vi "FRC Color Processing RetroTape Example.vi"() -> ()   [LabVIEW 2019]
uses:
  <vilib>/Rock Robotics/Network Tables/NT Event Type.ctl
  <vilib>/Rock Robotics/Network Tables/Protocol Operations.ctl
  <vilib>/Rock Robotics/Network Tables/Field Data.ctl
  <vilib>/Rock Robotics/Network Tables/Field Type.ctl
  <vilib>/Rock Robotics/Network Tables/Sequence.ctl
  <vilib>/vision/NI_Vision_Development_Module.lvlib
panel:
  in  "Tab Control":enum32{"Mask", "Post Processed"}(tab)=enum."Post Processed"
  out "Mask":T1(plugin-control)
  in  "LED Color Range":T2={"Hue"={103.0, 151.0}, "Sat"={216.98804569244385, 255.0}, "Val"={201.0, 249.0}} {"Hue" scale=0.0..255.0 scale format="%#_3g"}
  in  "Color Mode":u16(ring)=2 items=["RGB", "HSL", "HSV", "HSI"]
  in  "Std Devs":cluster{"H":dbl, "S":dbl, "V":dbl}={"H"=6.0, "S"=6.0, "V"=6.0}
  out "Offset Angle":dbl=-14.437499999999998 format="%.1f"
  out "Fps Processing":dbl=128.6646791248816 format="%#.0f"
  out "Results":T3(array[cluster])=[{"diameter points"={"first point"={"x"=290.0, "y"=32.0}, "projected point"={"x"=196.0, "y"=45.0}}, "Normalized Center"={"x"=-0.24062499999999998, "y"=-0.7861111111111111}, "Overall Score"=94.92498623274359, "Area Score"=96.95566094203232, "Moment Score"=88.10546356152027, "Aspect Score"=99.71383419467818, "Distance (ft)"=13.68022905002843, "Upper Goal"=TRUE}] {"Normalized Center"."x" format="%#_2g"; "Normalized Center"."y" format="%#_2g"; "Overall Score" format="%#_2g"; "Distance (ft)" format="%#_3g"; "Area Score" format="%#_2g"; "Moment Score" format="%#_2g"; "Aspect Score" format="%#_2g"}
  in  "Exit":bool
  out "Loop Time":dbl=7.76519775390625 format="%0.2f"
  in  "Field of view":dbl=170.0 format="%#_13g"
  out "Processed":T1(plugin-control)
  in  "Client Name":string="Vision"
  in  "Update Time (ms)":i32=6
  in  "Server IP Address":string="roboRIO-141-FRC.local"
  # "Scores"
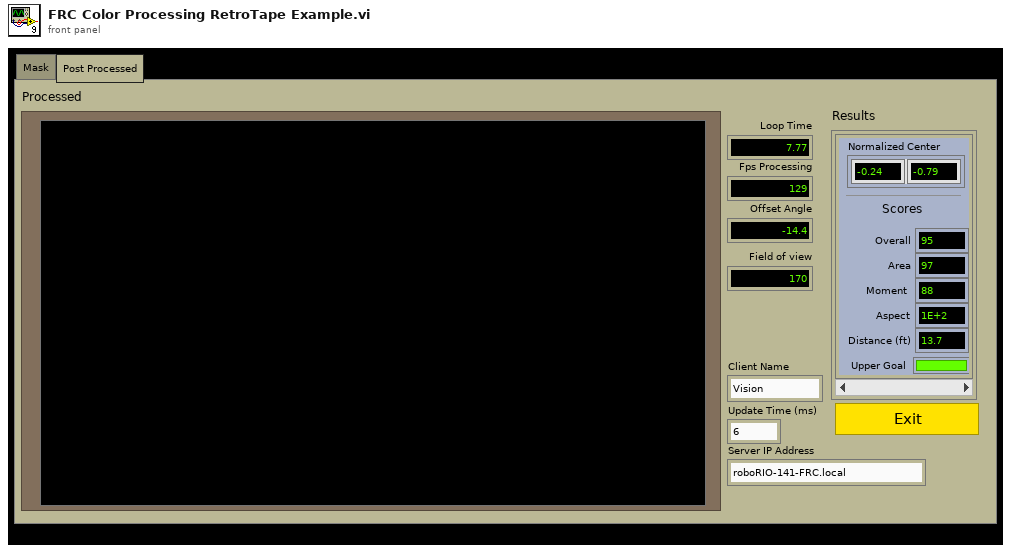
[diagram p1: front panel]
types:
  T1 = typedef "IMAQ Image.ctl" = refnum<image>
  T2 = cluster{"Hue":cluster{dbl, dbl}, "Sat":cluster{dbl, dbl}, "Val":cluster{dbl, dbl}}
  T3 = cluster{"diameter points":cluster{"first point":cluster{"x":dbl, "y":dbl}, "projected point":cluster{"x":dbl, "y":dbl}}, "Normalized Center":cluster{"x":dbl, "y":dbl}, "Overall Score":dbl, "Area Score":dbl, "Moment Score":dbl, "Aspect Score":dbl, "Distance (ft)":dbl, "Upper Goal":bool}[]
  T4 = typedef "NT Event Type.ctl" = cluster{"Operation":T5, "Name":string, "Field Value":T6}
  T5 = typedef "Protocol Operations.ctl" = enum16{"Unknown", "Keep Alive", "Client Hello", "Version not supported", "Server Hello Complete", "Assign", "Update", "No Op", "Server Hello", "Client Hello Complete", "Update Flags", "Delete Entry", "Delete All", "RPC Exec", "RPC Response"}
  T6 = typedef "Field Data.ctl" = cluster{"Dbl":dbl, "String":string, "Type":T7, "Boolean":bool, "Sequence #":T8, "Flags":u8}
  T7 = typedef "Field Type.ctl" = enum8{"Invalid", "Bool", "Numeric", "String", "Raw", "Boolean Array", "Numeric Array", "String Array", "RPC"}
  T8 = typedef "Sequence.ctl" = u16
  T9 = typedef "Image Type" = u32
  T10 = typedef "Particle Parameters" = i32
  T11 = cluster{cluster{dbl, dbl}, cluster{dbl, dbl}, cluster{dbl, dbl}}
  T12 = typedef "Target Fields.ctl" = cluster{"diameter points":cluster{"first point":cluster{"x":dbl, "y":dbl}, "projected point":cluster{"x":dbl, "y":dbl}}, "normalized center":cluster{"x":dbl, "y":dbl}, "Overall Score":dbl, "Area Score":dbl, "Moment Score":dbl, "Aspect Score":dbl, "Distance (ft)":dbl, "Upper Goal":bool}
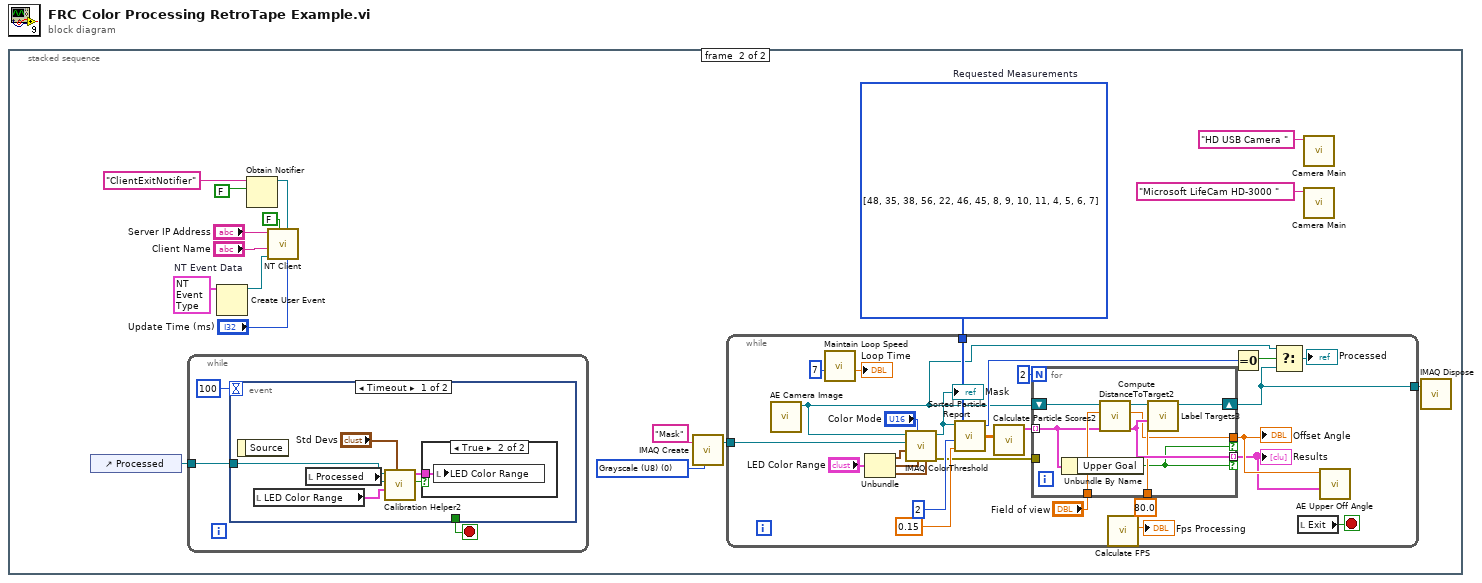
[diagram p0: block diagram]
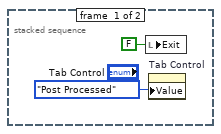
[diagram p2: hidden frame]
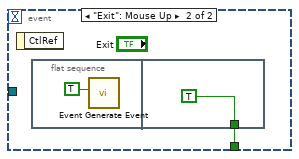
[diagram p4: hidden frame]
diagram:
  n1 = stacked-sequence {
    frame #0 {
      n2 = local write "Exit"(FALSE ("Exit")) -> ()
      n3 = property on="Tab Control" class="TabCtl (strict)"("Value"=enum32{"Mask", "Post Processed"}."Post Processed" ("Tab Control")) -> ()  [unwired: 2 in, 2 out]
    }
    frame #1 {
      w14 = T4 {"Operation"=enum."Assign", "Name"="", "Field Value"={"Dbl"=0.0, "String"="kjn", "Type"=enum."String", "Boolean"=FALSE, "Sequence #"=0, "Flags"=0}}  # NT Event Data
      w18 = T9 0 items=["Grayscale (U8)", "Grayscale (I16)", "Grayscale (SGL)", "Complex (CSG)", "RGB (U32)", "HSL (U32)", "RGB (U64)", "Grayscale (U16)"] ("Image Type")
      w19 = T10[] [48, 35, 38, 56, 22, 46, 45, 8, 9, 10, 11, 4, 5, 6, 7] items=["Center of Mass X", "Center of Mass Y", "First Pixel X", "First Pixel Y", "Bounding Rect Left", "Bounding Rect Top", "Bounding Rect Right", "Bounding Rect Bottom", "Max Feret Diameter Start X", "Max Feret Diameter Start Y", "Max Feret Diameter End X", "Max Feret Diameter End Y", "Max Horiz. Segment Length Left", "Max Horiz. Segment Length Right", "Max Horiz. Segment Length Row", "-", "Bounding Rect Width", "Bounding Rect Height", "Bounding Rect Diagonal", "Perimeter", "Convex Hull Perimeter", "Holes' Perimeter", "Max Feret Diameter", "Equivalent Ellipse Major Axis", "Equivalent Ellipse Minor Axis", "Equivalent Ellipse Minor Axis (Feret)", "Equivalent Rect Long Side", "Equivalent Rect Short Side", "Equivalent Rect Diagonal", "Equivalent Rect Short Side (Feret)", "Average Horiz. Segment Length", "Average Vert. Segment Length", "Hydraulic Radius", "Waddel Disk Diameter", "-", "Area", "Holes' Area", "Particle & Holes' Area", "Convex Hull Area", "Image Area", "-", "Number of Holes", "Number of Horiz. Segments", "Number of Vert. Segments", "-", "Orientation", "Max Feret Diameter Orientation", "-", "% Area/Image Area", "% Area/(Particle & Holes' Area)", "Ratio of Equivalent Ellipse Axes", "Ratio of Equivalent Rect Sides", "-", "Elongation Factor", "Compactness Factor", "Heywood Circularity Factor", "Type Factor", "-", "Sum X", "Sum Y", "Sum XX", "Sum XY", "Sum YY", "Sum XXX", "Sum XXY", "Sum XYY", "Sum YYY", "-", "Moment of Inertia XX", "Moment of Inertia XY", "Moment of Inertia YY", "Moment of Inertia XXX", "Moment of Inertia XXY", "Moment of Inertia XYY", "Moment of Inertia YYY", "Norm. Moment of Inertia XX", "Norm. Moment of Inertia XY", "Norm. Moment of Inertia YY", "Norm. Moment of Inertia XXX", "Norm. Moment of Inertia XXY", "Norm. Moment of Inertia XYY", "Norm. Moment of Inertia YYY", "Hu Moment 1", "Hu Moment 2", "Hu Moment 3", "Hu Moment 4", "Hu Moment 5", "Hu Moment 6", "Hu Moment 7"]  # Requested Measurements
      n4 = control-ref of="Processed"() -> (w3:refnum<vi>)
      n5 = while {
        tunnel: w3 -> [w22]
        stop <- w21 stop-if-true
        n6 = event shown="[0] Timeout" {
          selector: _ -> [_ _]
          dyn-events: _ -> [_ _]
          timeout: 100 -> [_ _]
          tunnel: w22 -> [w24 _]
          tunnel: [_ w30] -> w21
          event Timeout {
            n7 = event-data() -> ()  [unwired: 1 in, 1 out]
            n8 = local read "LED Color Range"() -> (w23:T2)
            n9 = local read "Processed"() -> (w25:T1)
            n10 = call "Calibration Helper2.vi"("Std Devs"="Std Devs", "Color Components"=w23, "Image"=w25, "Image Ctl Refnum"=w24) -> ("Changed"=w28:bool, "output color"=w27:T11)  [unwired: 6 in]
            n11 = case shown="True" w28 {
              tunnel: w27 -> [_ w29]
              frame False {
              }
              frame True {
                n12 = local write "LED Color Range"(w29) -> ()
              }
            }
          }
          event "Exit": Mouse Up {
            n13 = event-data() -> ()  [unwired: 1 in, 1 out]
            n14 = flat-sequence {
              tunnel: [TRUE] -> w30
              frame #0 {
                n15 = call "Event Generate Event.vi"("Exit"=TRUE) -> ()  [unwired: 11 in]
              }
              frame #1 {
              }
            }
          }
        }
      }
      n16 = Create User Event(user event datatype=w14) -> (user event=w8:refnum<user-event>)  [unwired: 1 in, 1 out]
      n17 = Obtain Notifier(name (unnamed)="ClientExitNotifier", notification data type=FALSE ("Automatic restart")) -> (notifier out=w10:refnum<notifier>)  [unwired: 2 in, 2 out]
      n18 = call <vilib>:"NT Client.vi"("Update Time"="Update Time (ms)", "Cancel Ref"=w10, "Automatic restart"=FALSE, "user event ref"=w8, "Client Name"="Client Name", "Server IP Address"="Server IP Address") -> ()  [unwired: 6 in]
      n19 = call "IMAQ Create"("Image Name"="Mask", "Image Type"=w18) -> ("New Image"=w16:T1)  [unwired: 2 in, 2 out]
      n20 = while {
        tunnel: w19 -> [w59]
        tunnel: w16 -> [w55]
        tunnel: [w37] -> w15
        stop <- w46 stop-if-true
        n21 = call "AE Camera Image.vi"() -> ("Upper Image out"=w34:T1)  [unwired: 11 in]
        n22 = call "Maintain Loop Speed.vi"("setpoint (msec)"=7) -> ("Loop Time"=→"Loop Time":dbl)  [unwired: 10 in]
        n23 = Unbundle("LED Color Range") -> ("Hue"=w56:cluster{dbl, dbl}, "Sat"=w58:cluster{dbl, dbl}, "Val"=w57:cluster{dbl, dbl})
        n24 = call "IMAQ ColorThreshold"("Blue or Luma or Val or Inten Range"=w57, "Green or Sat Range"=w58, "Color Mode"="Color Mode", "Red or Hue Range"=w56, "Image Dst"=w55, "Image Src"=w34) -> ("error out"=w48:errorcluster, "Image Dst Out"=w33:T1)  [unwired: 4 in]
        "Mask" <- w33
        n25 = call "Sorted Particle Report.vi"("Min Area Size %"=0.15 ("Size Limit %"), "Particle Count Limit"=2 ("Particle Count"), "Pixel Measurements"=w59, "Image in"=w33) -> ("Sorted Data"=w51:dbl[][], "Particles"=w42:i32)  [unwired: 1 out]
        n26 = call "Calculate Particle Scores2.vi"("Sorted Data"=w51) -> ("Scores"=w50:T12[])  [unwired: 10 in]
        n27 = for {
          N: 2 -> [_]
          tunnel: w50 -> [w62] mode=indexing
          tunnel: [w65] -> w38 mode=indexing if=w60
          tunnel: [w61] -> w39 if=w60
          tunnel: 80.0 ("Score Threshold %") -> [w64]
          tunnel: w48 -> [_]
          tunnel: "Field of view" -> [w63]
          shift-right: [w68] -> w37
          shift-left: w34 -> [w67]
          n28 = Unbundle By Name(w62) -> ("Upper Goal"=w60:bool)
          n29 = call "Compute DistanceToTarget2.vi"("results"=w62, "Field of view"=w63, "Image Src"=w67) -> ("results out"=w65:T12, "Offset Angle"=w61:dbl, "Image Dst Out"=w66:T1)  [unwired: 6 in]
          n30 = call "Label Targets3.vi"("Score Threshold"=w64, "results"=w65, "Image in"=w66) -> ("Image out"=w68:T1)  [unwired: 8 in]
        }
        "Results" <- w38
        "Offset Angle" <- w39
        n31 = call "Calculate FPS.vi"() -> ("Fps"=→"Fps Processing":dbl)  [unwired: 11 in]
        n32 = Equal To 0?(x=w42) -> (x = 0?=w35:bool)
        n33 = Select(t=w34, s=w35, f=w37) -> (s? t:f=→"Processed":T1)
        n34 = local read "Exit"() -> (w46:bool)
        n35 = call "AE Upper Off Angle.vi"("Results 2"=w38, "Upper Off Angle"=w39) -> ()  [unwired: 9 in, 1 out]
      }
      n36 = call "Camera Main.vi"("Camera Name"="HD USB Camera " ("y")) -> ()  [unwired: 11 in]
      n37 = call "Camera Main.vi"("Camera Name"="Microsoft LifeCam HD-3000 " ("y")) -> ()  [unwired: 11 in]
      n38 = call "IMAQ Dispose"("Image"=w15) -> ()  [unwired: 5 in, 1 out]
    }
  }
